vi "VisaBasicForS3.vi"(1 "VISA resource name":refnum<visa-resource-name>, 2 "Cmd":string, 3 "TimeOut":bool=TRUE, 4 "Time(0.1)":u32=10, 5 "error in (no error)":errorcluster, 8 "VisaAction":enum16{"Open", "Send", "Recieve", "Close"}(ring)) -> (16 "read string":string, 19 "error out":errorcluster)   [LabVIEW 2019]
uses:
  <vilib>/Instr/_visa.llb/VISA Configure Serial Port (Instr).vi
  LLB/Commonly VI.lvlib
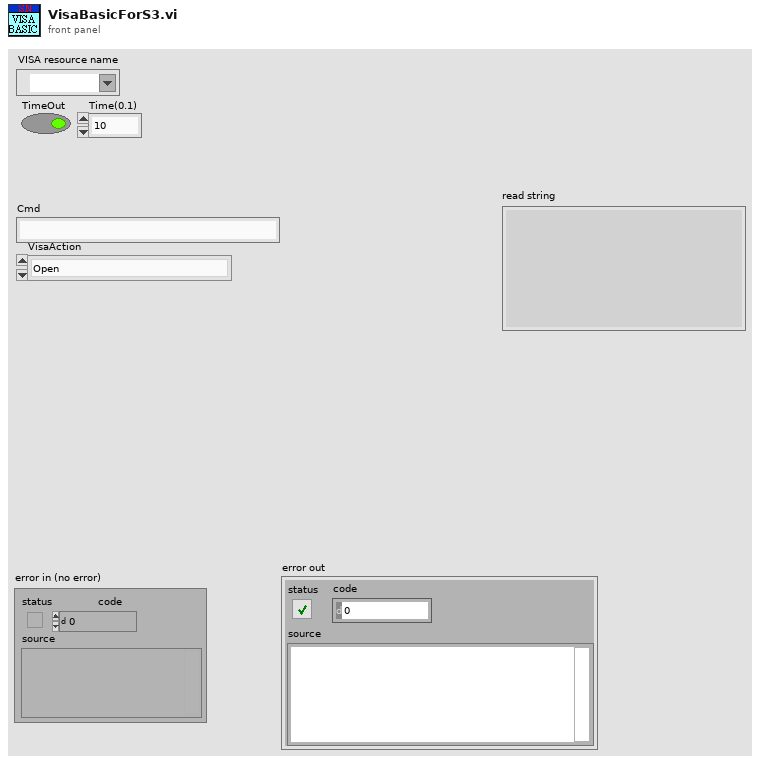
[diagram p1: front panel]
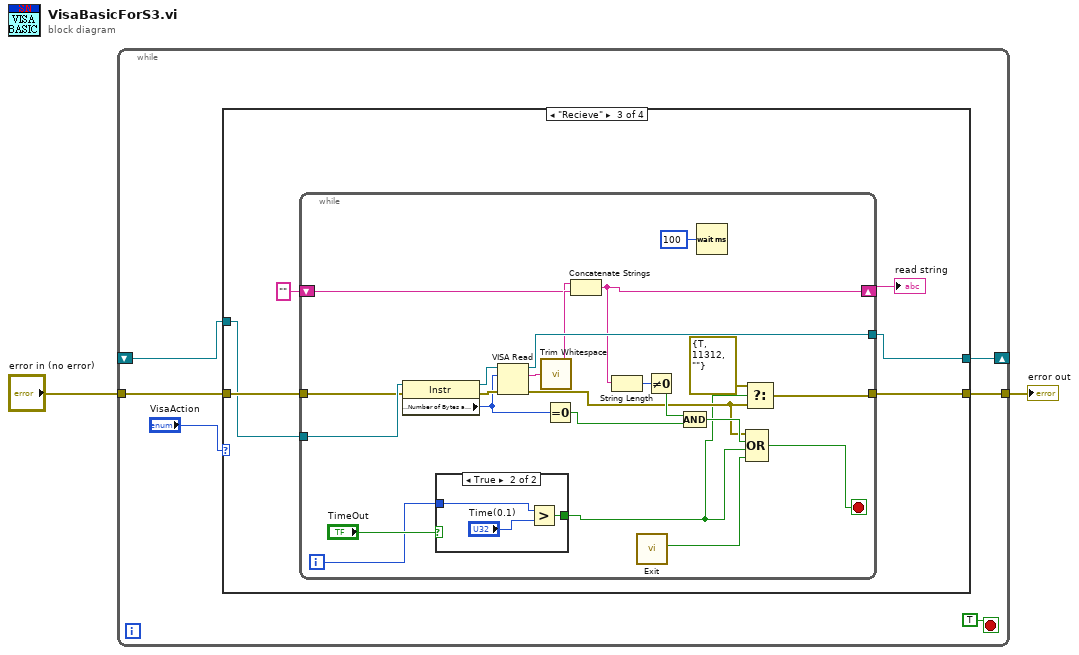
[diagram p0: block diagram]
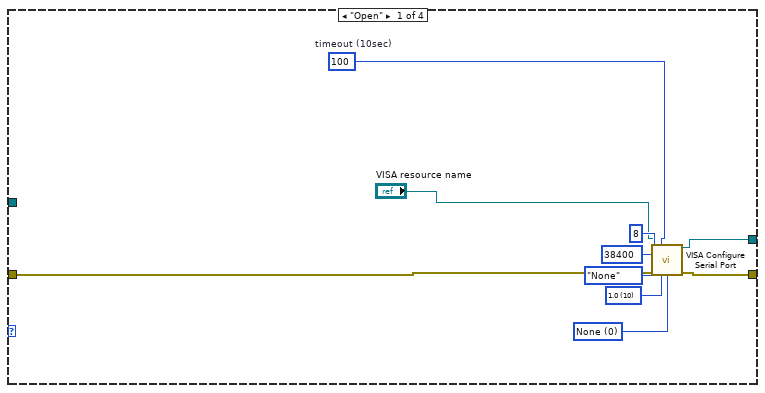
[diagram p2: hidden frame]
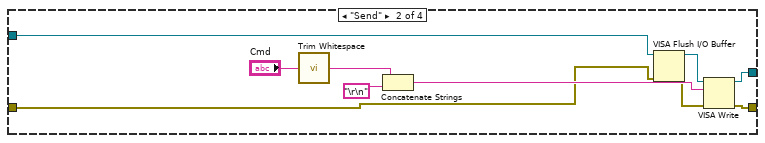
[diagram p3: hidden frame]
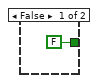
[diagram p4: hidden frame]
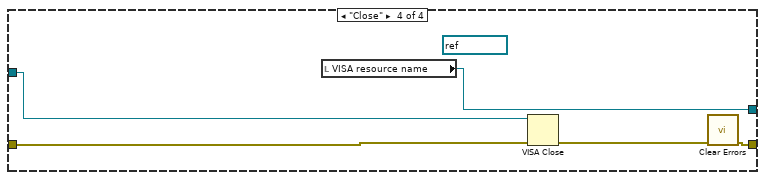
[diagram p5: hidden frame]
diagram:
  n1 = while {
    tunnel: "error in (no error)" -> [w6]
    tunnel: [w7] -> w2
    shift-right: [w4] -> _
    shift-left: _ -> [w3]
    stop <- TRUE stop-if-true
    n2 = case shown="\"Recieve\"" "VisaAction" {
      tunnel: [w18 w28 w33 w63] -> w7
      tunnel: w6 -> [w17 w19 w34 w65]
      tunnel: w3 -> [_ w20 w30 w64]
      tunnel: [w10 w23 w29 w62] -> w4
      frame "Open" {
        w12 = u16 0 items=["None", "XON/XOFF", "RTS/CTS", "XON/XOFF & RTS/CTS", "DTR/DSR", "XON/XOFF & DTR/DSR"] ("flow control (0:none)")
        w13 = u16 10 items=["1.0"=10, "1.5"=15, "2.0"=20] ("stop bits (10: 1 bit)")
        w16 = u32 100  # timeout (10sec)
        n3 = call-poly "VISA Configure Serial Port"("VISA resource name"="VISA resource name", "timeout (10sec)"=w16, "baud rate (9600)"=u32 38400, "data bits (8)"=u16 8, "parity (0:none)"=enum16{"None", "Odd", "Even", "Mark", "Space"}."None", "error in (no error)"=w17, "stop bits (10: 1 bit)"=w13, "flow control (0:none)"=w12) -> ("VISA resource name out"=w10:refnum<visa-resource-name>, "error out"=w18:errorcluster)  [unwired: 1 in, 5 out]
      }
      frame "Send" {
        n4 = call <vilib>:"Trim Whitespace.vi"("string"="Cmd") -> ("trimmed string"=w24:string)  [unwired: 1 in]
        n5 = Concatenate Strings(w24, "\r\n") -> (w25:string)
        n6 = VISA Flush I/O Buffer(VISA resource name=w20, error in (no error)=w19) -> (VISA resource name out=w21:refnum<visa-resource-name>, error out=w22:errorcluster)  [unwired: 1 in]
        n7 = VISA Write(VISA resource name=w21, write buffer=w25, error in (no error)=w22) -> (VISA resource name out=w23:refnum<visa-resource-name>, error out=w28:errorcluster)  [unwired: 1 out]
      }
      frame "Recieve" {
        n8 = while {
          tunnel: w30 -> [w55]
          tunnel: w34 -> [w54]
          tunnel: [w53] -> w29
          tunnel: [w48] -> w33
          shift-right: [w45] -> w32
          shift-left: "" ("trimmed string") -> [w51]
          i -> [w36]
          stop <- w49 stop-if-true
          n9 = property class="Instr"(reference=w55, error in=w54) -> (reference out=w56:refnum<visa-resource-name>, error out=w57:errorcluster, "Serial Settings:Number of Bytes at Serial Port"=w37:u32)
          n10 = case shown="True" "TimeOut" {
            tunnel: w36 -> [_ w61]
            tunnel: [FALSE w59] -> w35
            frame False {
            }
            frame True {
              n11 = Greater?(x=w61, y="Time(0.1)") -> (0:w59:bool)
            }
          }
          n12 = VISA Read(VISA resource name=w56, byte count=w37, error in (no error)=w57) -> (VISA resource name out=w53:refnum<visa-resource-name>, read buffer=w39:string, error out=w41:errorcluster)  [unwired: 1 out]
          n13 = call <vilib>:"Trim Whitespace.vi"("string"=w39) -> ("trimmed string"=w52:string)  [unwired: 1 in]
          n14 = Equal To 0?(x=w37) -> (x = 0?=w46:bool)
          n15 = Concatenate Strings(w51, w52) -> (w45:string)
          n16 = String Length(string=w45) -> (length=w44:i32)
          n17 = call "Exit.vi"() -> ("ExitOut"=w40:bool)  [unwired: 11 in]
          n18 = Not Equal To 0?(x=w44) -> (x != 0?=w43:bool)
          n19 = Compound Arithmetic op=AND(w43, w46) -> (w42:bool)
          n20 = Wait (ms)(milliseconds to wait=u32 100) -> ()  [unwired: 1 out]
          n21 = Select(t=errorcluster {"status"=TRUE, "code"=11312, "source"=""}, s=w35, f=w41) -> (s? t:f=w48:errorcluster)
          n22 = Compound Arithmetic op=OR(w41, w42, w35, w40) -> (w49:bool)
        }
        "read string" <- w32
      }
      frame "Close" {
        (unwired) refnum<visa-resource-name> "COM3" ("VISA resource name out")
        n23 = local read "VISA resource name"() -> (w62:refnum<visa-resource-name>)
        n24 = VISA Close(VISA resource name=w64, error in (no error)=w65) -> (error out=w66:errorcluster)
        n25 = call <vilib>:"Clear Errors.vi"("error in (no error)"=w66) -> ("error out"=w63:errorcluster)  [unwired: 5 in, 1 out]
      }
    }
  }
  "error out" <- w2
